vi "SENS_SEGM_FREQ_START.vi"(0 "VISA IN":refnum<visa-resource-name>, 1 "Segment":i32, 2 "Frq. Start(Hz)":i32, 5 "error in":errorcluster, 7 "Channel":i32) -> (14 "VISA Out":refnum<visa-resource-name>, 19 "error out":errorcluster)   [LabVIEW 2018, in "PNA-X.lvlib"]
doc: "SENSe<cnum>:SEGMent<snum>:FREQuency:START <num> \n(Read-Write) Sets the Start Frequency for the specified sweep segment. \nNotes \nAll other segment Start and Stop Frequency values that are larger than this frequency are changed to \nthis frequency. \nTo return the start and stop frequency of the entire sweep (all segments), Use SENS:FREQ:STARt? \nand SENS:FREQ:STOP? \nParameters \n<cnum> Any existing channel number. If unspecified, value is set to 1 \n<snum> Segment number to modify. Choose any existing segment number. \n<num> Start Frequency in Hz. Choose any number between the minimum and \nmaximum frequency of the analyzer. \nNote: This command will accept MIN or MAX instead of a numeric parameter. \n1809\n\nSee SCPI Syntax for more information. \nExamples SENS:SEGM:FREQ:STAR 1MHZ \nsense2:segment2:frequency:start minimum \nQuery Syntax SENSe<cnum>:SEGMent<snum>:FREQuency:STARt? \nReturn Type Numeric \nDefault Stop Frequency of the previous segment. If first segment, start frequency of the \nanalyzer."
uses:
  PNA-X.lvlib
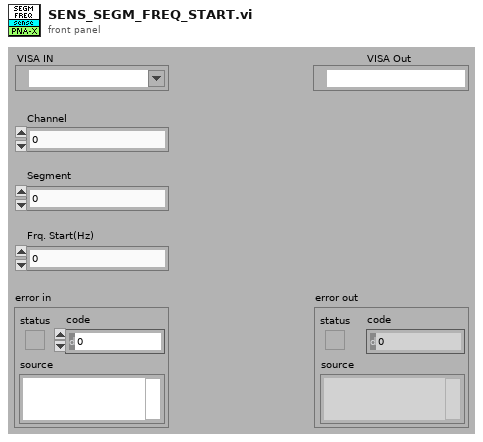
[diagram p1: front panel]
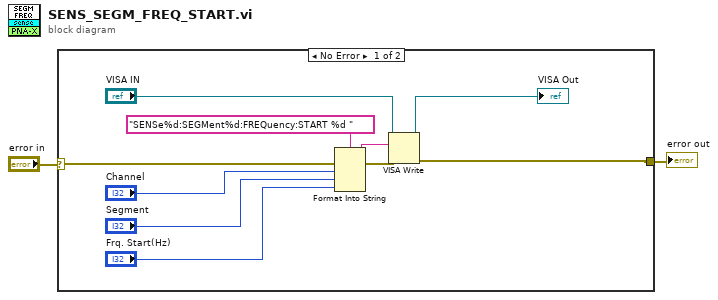
[diagram p0: block diagram]
diagram:
  n1 = case shown="No Error" "error in" {
    selector: "error in" -> [w12 w13]
    tunnel: [w7 w13] -> w1
    frame No Error {
      n2 = Format Into String(format string="SENSe%d:SEGMent%d:FREQuency:START %d " ("Cmdline"), error in=w12, "Channel", "Segment", "Frq. Start(Hz)") -> (resulting string=w10:string, error out=w11:errorcluster)  [unwired: 1 in]
      n3 = VISA Write(VISA resource name="VISA IN", write buffer=w10, error in (no error)=w11) -> (VISA resource name out=→"VISA Out":refnum<visa-resource-name>, error out=w7:errorcluster)  [unwired: 1 out]
    }
    frame Error {
    }
  }
  "error out" <- w1
